vi "Is MessageQ Empty.vi"(8 "error in (no error)":errorcluster, 11 "Process in":refnum<class "Process.lvclass">) -> (0 "error out":errorcluster, 2 "is Empty ?":bool, 3 "Process out":refnum<class "Process.lvclass">)   [LabVIEW 2019, in "TimingDRV Engine.lvlib" / "Process.lvclass"]
uses:
  Process.lvclass
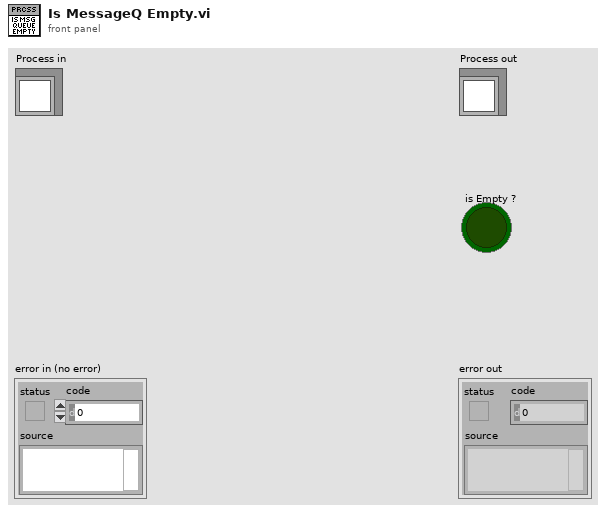
[diagram p1: front panel]
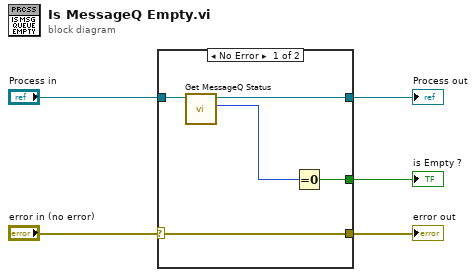
[diagram p0: block diagram]
diagram:
  n1 = case shown="No Error" "error in (no error)" {
    selector: "error in (no error)" -> [w10 w12]
    tunnel: [w10 w12] -> w4
    tunnel: [w7 w11] -> w2
    tunnel: "Process in" -> [w9 w11]
    tunnel: [w6 _] -> w1
    frame No Error {
      n2 = call "Get MessageQ Status.vi"("Process in"=w9) -> ("# elements in MessageQ"=w8:i32, "Process out"=w7:refnum<class "Process.lvclass">)  [unwired: 7 in, 2 out]
      n3 = Equal To 0?(x=w8) -> (x = 0?=w6:bool)
    }
    frame Error {
    }
  }
  "error out" <- w4
  "Process out" <- w2
  "is Empty ?" <- w1
